vi "信号去噪.vi"(3 "字符串":string, 4 "数值":i32, 5 "文件路径（输入）":path) -> (0 "去噪后数据输出":dbl[][](array[numeric]), 2 "去噪后波形图（输出）":dbl[][](graph))   [LabVIEW 2018]
uses:
  <vilib>/Utility/error.llb/whitespace.ctl
panel:
  in  "noisy1.IClass1":refnum<k7>
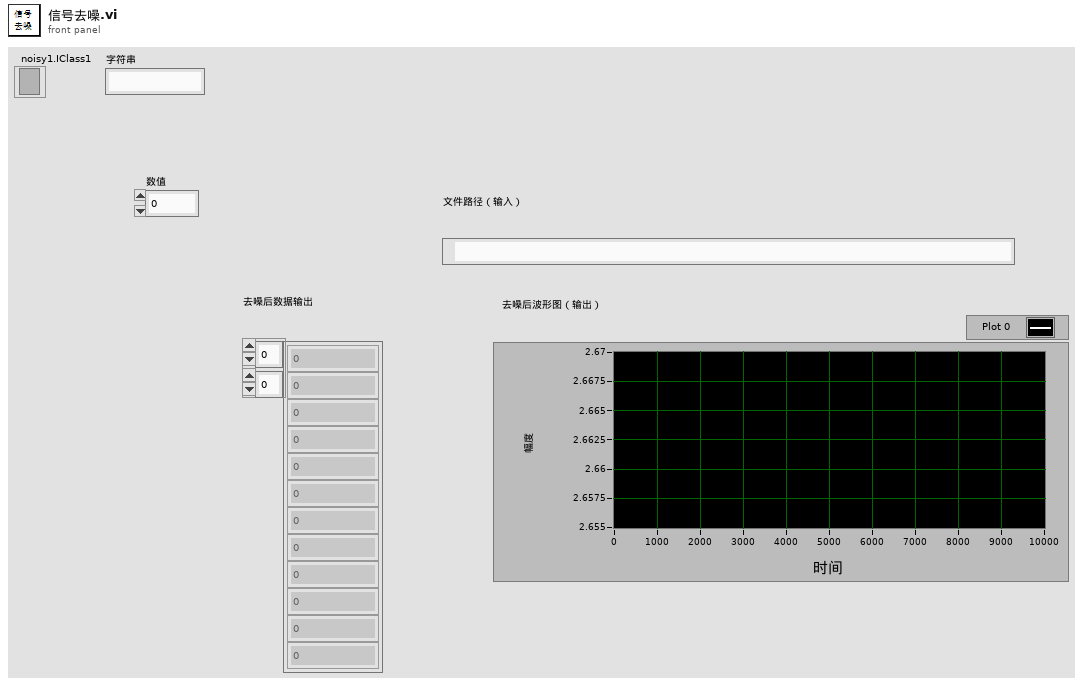
[diagram p1: front panel]
types:
  T1 = typedef "whitespace.ctl" = u16
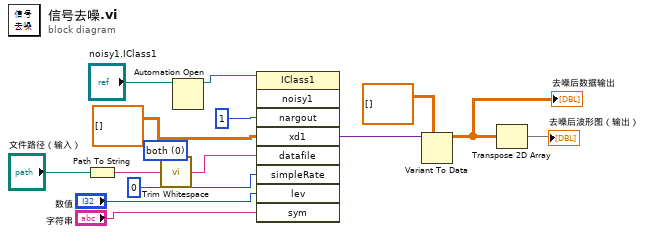
[diagram p0: block diagram]
diagram:
  w7 = T1 0 items=["both", "start of string", "end of string"] ("location (both)")
  n1 = Path To String(path="文件路径（输入）") -> (string=w6:string)
  n2 = call <vilib>:"Trim Whitespace.vi"("string"=w6, "location (both)"=w7) -> ("trimmed string"=w5:string)
  n3 = Automation Open(Automation Refnum="noisy1.IClass1") -> (Automation Refnum=w14:refnum<k7>)  [unwired: 3 in, 1 out]
  n4 = invoke class="IClass1" method="noisy1"(reference=w14, "nargout"=1, "xd1"=dbl[][] [] ("type"), "datafile"=w5, "simpleRate"=0, "lev"="数值", "sym"="字符串") -> ("xd1"=w13:variant)  [unwired: 2 in, 8 out]
  n5 = Variant To Data(type=dbl[][] [], Variant=w13) -> (data=w8:dbl[][])  [unwired: 1 in, 1 out]
  "去噪后数据输出" <- w8
  n6 = Transpose 2D Array(2D array=w8) -> (transposed array=→"去噪后波形图（输出）":dbl[][])
